vi "lift auto.vi"(1 "Current Setpoint":dbl, 2 "Auto GoTo Location":dbl, 4 "Index":T1) -> (0 "Setpoint":dbl)   [LabVIEW 2014]
uses:
  typedefs/lift/lift command.ctl
  global variables/devrefs.vi
panel:
  # "For Autonomous mode only"
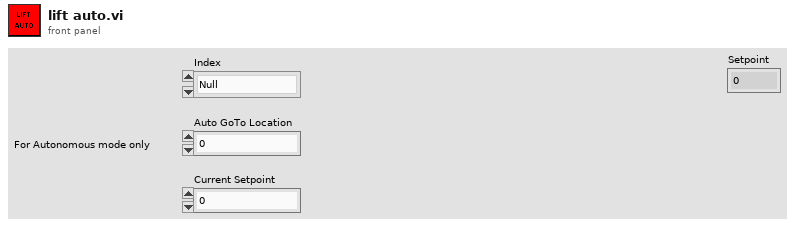
[diagram p1: front panel]
types:
  T1 = typedef "lift command.ctl" = enum16{"Null", "Index Up", "Index Down", "Go To Home", "Cap 4 Stack", "Container Index Up", "Container Index Down", "Autonomous"}
  T2 = typedef "subStates.ctl" = enum16{"null", "wait", "driver control", "auto", "manual override", "hold position", "rotate", "test", "end"}
  T3 = typedef "WPI_EncoderDevRef.ctl" = cluster{"DevStatus":errorcluster, "EncoderIndex":T4, "CounterIndex":T5, "DistancePerCount":dbl, "Decoding Type":T6}
  T4 = typedef "FPGA_EncoderIdx.ctl" = enum8{"Enc 0", "Enc 1", "Enc 2", "Enc 3", "Enc 4", "Enc 5", "Enc 6", "Enc 7", "Invalid"}
  T5 = typedef "FPGA_CounterCtrSystemIndex.ctl" = enum8{"Ctr 0", "Ctr 1", "Ctr 2", "Ctr 3", "Ctr 4", "Ctr 5", "Ctr 6", "Ctr 7", "Invalid"}
  T6 = typedef "WPI_EncoderType.ctl" = enum16{"1x", "2x", "4x"}
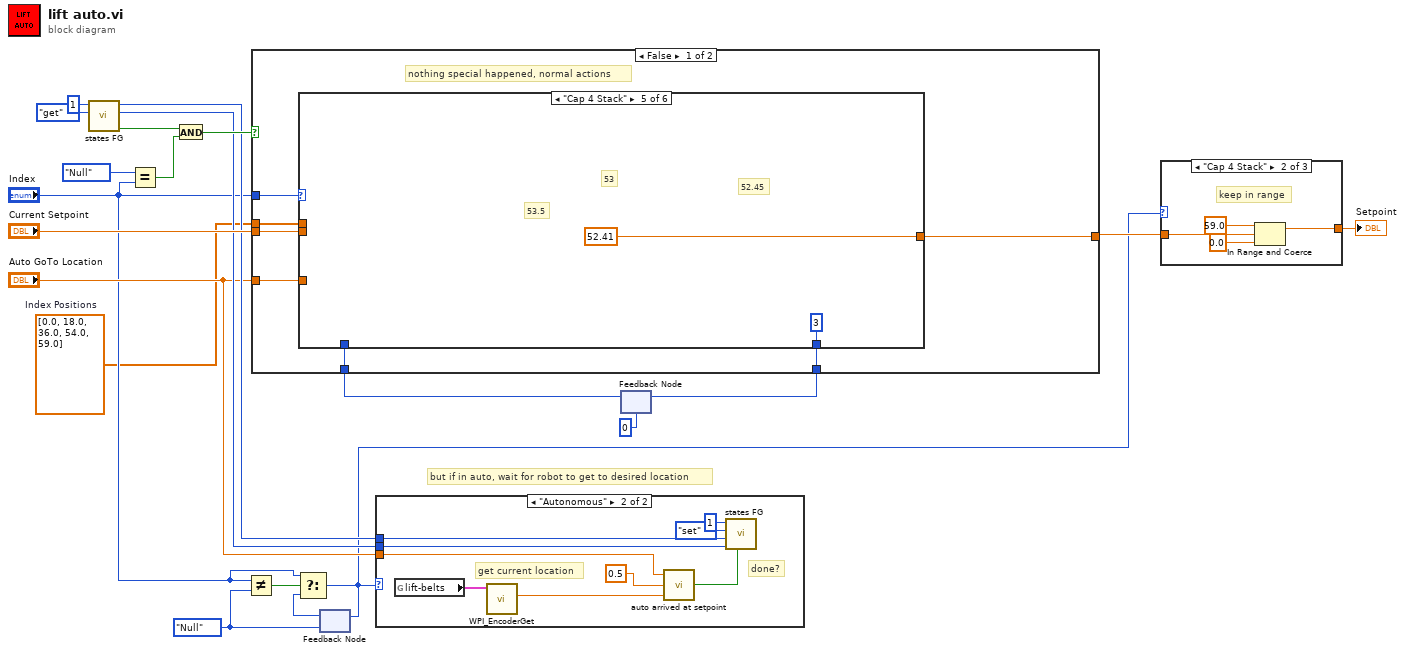
[diagram p0: block diagram]
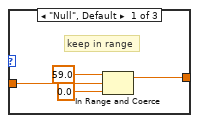
[diagram p3: hidden frame]
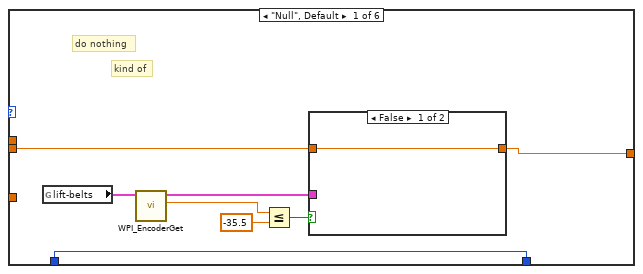
[diagram p5: hidden frame]
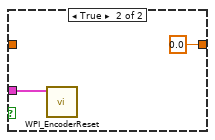
[diagram p6: hidden frame]
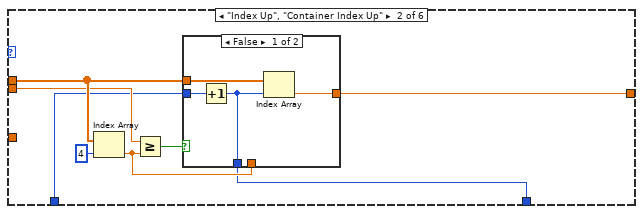
[diagram p7: hidden frame]
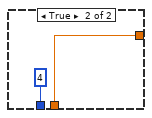
[diagram p8: hidden frame]
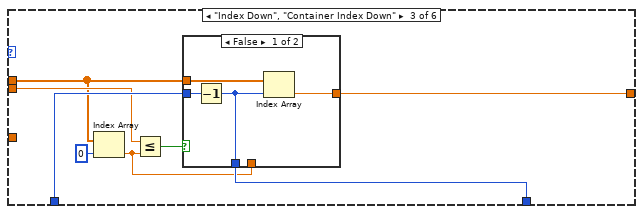
[diagram p9: hidden frame]
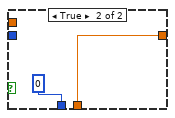
[diagram p10: hidden frame]
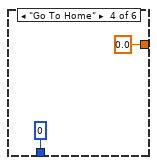
[diagram p11: hidden frame]
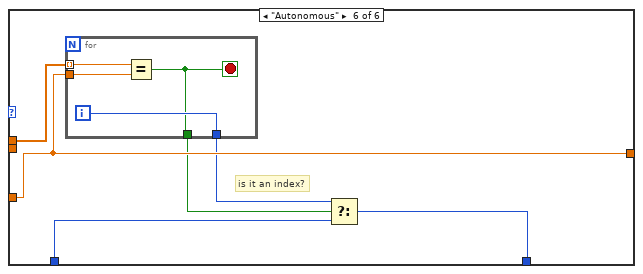
[diagram p12: hidden frame]
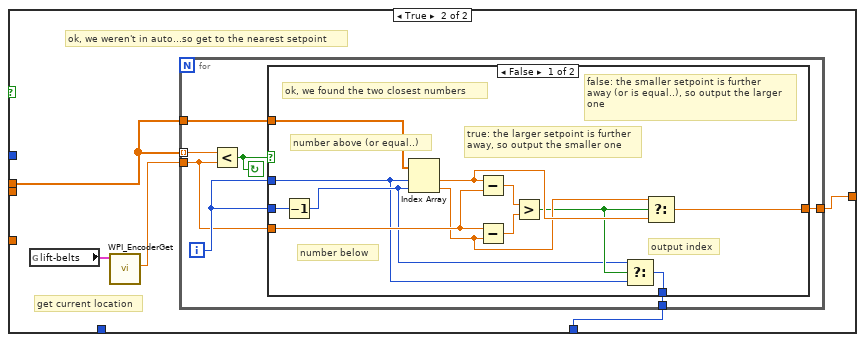
[diagram p13: hidden frame]
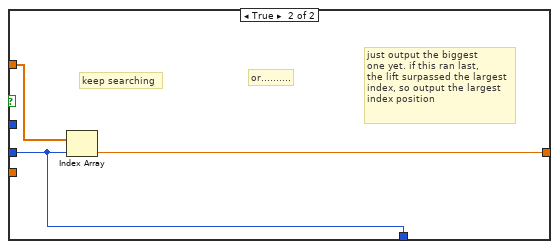
[diagram p14: hidden frame]
diagram:
  w4 = dbl[] [0.0, 18.0, 36.0, 54.0, 59.0]  # Index Positions
  w6 = lift_command."Null" ("Lift Command")
  # "but if in auto, wait for robot to get to desired location"
  n1 = call "states FG.vi"("menu (get)"=enum16{"set", "get"}."get", "Loop ID"=1) -> ("first call?"=w19:bool, "state # out"=w11:i32, "subState out"=w12:T2)  [unwired: 6 in, 1 out]
  n2 = Equal?(x=lift_command."Null", y="Index") -> (x = y?=w15:bool)
  n3 = And(x=w19, y=w15) -> (x .and. y?=w16:bool)
  n4 = Not Equal?(x="Index", y=w6) -> (x != y?=w9:bool)
  n5 = feedback #1(w6) -> (w8:T1)
  n6 = Select(t="Index", s=w9, f=w8) -> (s? t:f=w5:T1)
  n7 = feedback-in #1(w5) -> ()
  n8 = case shown="\"Autonomous\"" w5 {
    tunnel: w12 -> [_ w28]
    tunnel: w11 -> [_ w27]
    tunnel: "Auto GoTo Location" -> [_ w26]
    frame Default {
      # "not in auto"
    }
    frame "Autonomous" {
      # "done?"
      # "get current location"
      n9 = global read "devrefs.vi" "lift-belts"() -> (w23:T3)
      n10 = call <vilib>:"WPI_EncoderGet.vi"("EncoderDevRef"=w23) -> ("Distance"=w22:dbl)  [unwired: 5 in, 5 out]
      n11 = call "auto arrived at setpoint.vi"("Encoder Distance"=w22, "Tolerance"=0.5, "Setpoint"=w26) -> ("At Location?"=w24:bool)
      n12 = call "states FG.vi"("exit in"=w24, "state # in"=w27, "subState in"=w28, "menu (get)"=enum16{"set", "get"}."set", "Loop ID"=1) -> ()  [unwired: 3 in, 4 out]
    }
  }
  n13 = feedback #2(0) -> (w2:i32)
  n14 = case shown="False" w16 {
    tunnel: "Index" -> [w37 _]
    tunnel: "Current Setpoint" -> [w36 _]
    tunnel: [w35 w93] -> w14
    tunnel: "Auto GoTo Location" -> [w34 _]
    tunnel: w4 -> [w33 w92]
    tunnel: w2 -> [w32 _]
    tunnel: [w31 w91] -> w1
    frame False {
      # "nothing special happened, normal actions"
      n15 = case shown="\"Cap 4 Stack\"" w37 {
        tunnel: w36 -> [w43 w51 w68 _ _ _]
        tunnel: [w42 w53 w69 0.0 ("Current Setpoint") 52.41 ("Current Setpoint") w85] -> w35
        tunnel: w34 -> [_ _ _ _ _ w85]
        tunnel: w33 -> [_ w52 w66 _ _ w86]
        tunnel: w32 -> [w38 w50 w70 _ _ w81]
        tunnel: [w38 w49 w64 0 3 w82] -> w31
        frame "Null", Default {
          # "kind of"
          # "do nothing"
          n16 = global read "devrefs.vi" "lift-belts"() -> (w41:T3)
          n17 = call <vilib>:"WPI_EncoderGet.vi"("EncoderDevRef"=w41) -> ("Distance"=w39:dbl, "EncoderDevRef"=w40:T3)  [unwired: 5 in, 4 out]
          n18 = Less Or Equal?(x=w39, y=-35.5) -> (x <= y?=w44:bool)
          n19 = case shown="False" w44 {
            tunnel: w40 -> [_ w48]
            tunnel: [w46 0.0 ("Current Setpoint")] -> w42
            tunnel: w43 -> [w46 _]
            frame False {
            }
            frame True {
              n20 = call <vilib>:"WPI_EncoderReset.vi"("EncoderDevRef"=w48) -> ()  [unwired: 9 in, 2 out]
            }
          }
        }
        frame "Index Up", "Container Index Up" {
          n21 = Index Array(array=w52, index=4) -> (element=w54:dbl)
          n22 = Greater Or Equal?(x=w51, y=w54) -> (x >= y?=w55:bool)
          n23 = case shown="False" w55 {
            tunnel: w50 -> [w58 _]
            tunnel: [w60 w61] -> w53
            tunnel: w52 -> [w59 _]
            tunnel: [w57 4] -> w49
            tunnel: w54 -> [_ w61]
            frame False {
              n24 = Increment(x=w58) -> (x+1=w57:i32)
              n25 = Index Array(array=w59, index=w57) -> (element=w60:dbl)
            }
            frame True {
            }
          }
        }
        frame "Index Down", "Container Index Down" {
          n26 = Index Array(array=w66, index=0) -> (element=w63:dbl)
          n27 = Less Or Equal?(x=w68, y=w63) -> (x <= y?=w65:bool)
          n28 = case shown="False" w65 {
            tunnel: w70 -> [w72 _]
            tunnel: [w74 w75] -> w69
            tunnel: w66 -> [w73 _]
            tunnel: [w71 0] -> w64
            tunnel: w63 -> [_ w75]
            frame False {
              n29 = Decrement(x=w72) -> (x-1=w71:i32)
              n30 = Index Array(array=w73, index=w71) -> (element=w74:dbl)
            }
            frame True {
            }
          }
        }
        frame "Go To Home" {
        }
        frame "Cap 4 Stack" {
          # "53.5"
          # "53"
          # "52.45"
        }
        frame "Autonomous" {
          # "is it an index?"
          n31 = for {
            tunnel: w86 -> [w90] mode=indexing
            tunnel: w85 -> [w89]
            tunnel: [w88] -> w83
            tunnel: [w87] -> w84
            i -> [w88]
            stop <- w87 stop-if-true
            n32 = Equal?(x=w90, y=w89) -> (x = y?=w87:bool)
          }
          n33 = Select(t=w83, s=w84, f=w81) -> (s? t:f=w82:i32)
        }
      }
    }
    frame True {
      # "get current location"
      # "ok, we weren't in auto...so get to the nearest setpoint"
      n34 = global read "devrefs.vi" "lift-belts"() -> (w95:T3)
      n35 = call <vilib>:"WPI_EncoderGet.vi"("EncoderDevRef"=w95) -> ("Distance"=w94:dbl)  [unwired: 5 in, 5 out]
      n36 = for {
        tunnel: w92 -> [w102] mode=indexing
        tunnel: w94 -> [w99]
        tunnel: w92 -> [w100]
        tunnel: [w98] -> w93
        tunnel: [w96] -> w91
        i -> [w101]
        stop <- w97 continue-if-true
        n37 = Less?(x=w102, y=w99) -> (x < y?=w97:bool)
        n38 = case shown="False" w97 {
          tunnel: w101 -> [w104 _]
          tunnel: w101 -> [w113 w115]
          tunnel: w100 -> [w114 w117]
          tunnel: w99 -> [w112 _]
          tunnel: [w107 w116] -> w98
          tunnel: [w103 w115] -> w96
          frame False {
            # "output index"
            # "false: the smaller setpoint is further\naway (or is equal..), so output the larger\none"
            # "true: the larger setpoint is further\naway, so output the smaller one"
            # "number above (or equal..)"
            # "number below"
            # "ok, we found the two closest numbers"
            n39 = Decrement(x=w113) -> (x-1=w105:i32)
            n40 = Index Array(array=w114, index #1=w104, index #2=w105) -> (element #1=w109:dbl, element #2=w108:dbl)
            n41 = Subtract(x=w109, y=w112) -> (x-y=w110:dbl)
            n42 = Subtract(x=w112, y=w108) -> (x-y=w111:dbl)
            n43 = Greater?(x=w110, y=w111) -> (0:w106:bool)
            n44 = Select(t=w105, s=w106, f=w104) -> (s? t:f=w103:i32)
            n45 = Select(t=w108, s=w106, f=w109) -> (s? t:f=w107:dbl)
          }
          frame True {
            # "or.........."
            # "just output the biggest\none yet. if this ran last, \nthe lift surpassed the largest\nindex, so output the largest\nindex position"
            # "keep searching"
            n46 = Index Array(array=w117, index=w115) -> (element=w116:dbl)
          }
        }
      }
    }
  }
  n47 = feedback-in #2(w1) -> ()
  n48 = case shown="\"Cap 4 Stack\"" w5 {
    tunnel: w14 -> [w119 w123 w126]
    tunnel: [w118 w122 w126] -> w13
    frame "Null", Default {
      # "keep in range"
      n49 = In Range and Coerce(upper limit=59.0, x=w119, lower limit=0.0) -> (coerced(x)=w118:dbl)  [unwired: 1 out]
    }
    frame "Cap 4 Stack" {
      # "keep in range"
      n50 = In Range and Coerce(upper limit=59.0, x=w123, lower limit=0.0) -> (coerced(x)=w122:dbl)  [unwired: 1 out]
    }
    frame "Autonomous" {
    }
  }
  "Setpoint" <- w13
